vi "Create Name.vi"(6 "Name":string, 8 "error in":errorcluster, 9 "Name Library File Path":path, 10 "Active Project":refnum<vi>) -> (0 "error out":errorcluster, 2 "Name":T1)   [LabVIEW 2020, in "_Rescript.lvlib" / "Msg.lvlib" / "Msg.lvclass"]
uses:
  Msg.lvclass
  Name.ctl
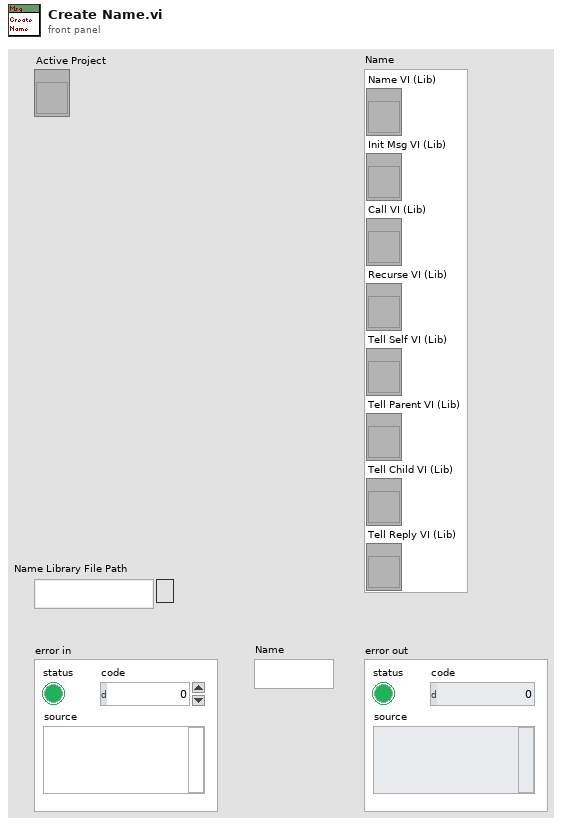
[diagram p1: front panel]
types:
  T1 = typedef "_Rescript.lvlib/Msg.lvlib/Msg.lvclass/Name.ctl" = cluster{"Name VI (Lib)":refnum<vi>, "Init Msg VI (Lib)":refnum<vi>, "Call VI (Lib)":refnum<vi>, "Recurse VI (Lib)":refnum<vi>, "Tell Self VI (Lib)":refnum<vi>, "Tell Parent VI (Lib)":refnum<vi>, "Tell Child VI (Lib)":refnum<vi>, "Tell Reply VI (Lib)":refnum<vi>}
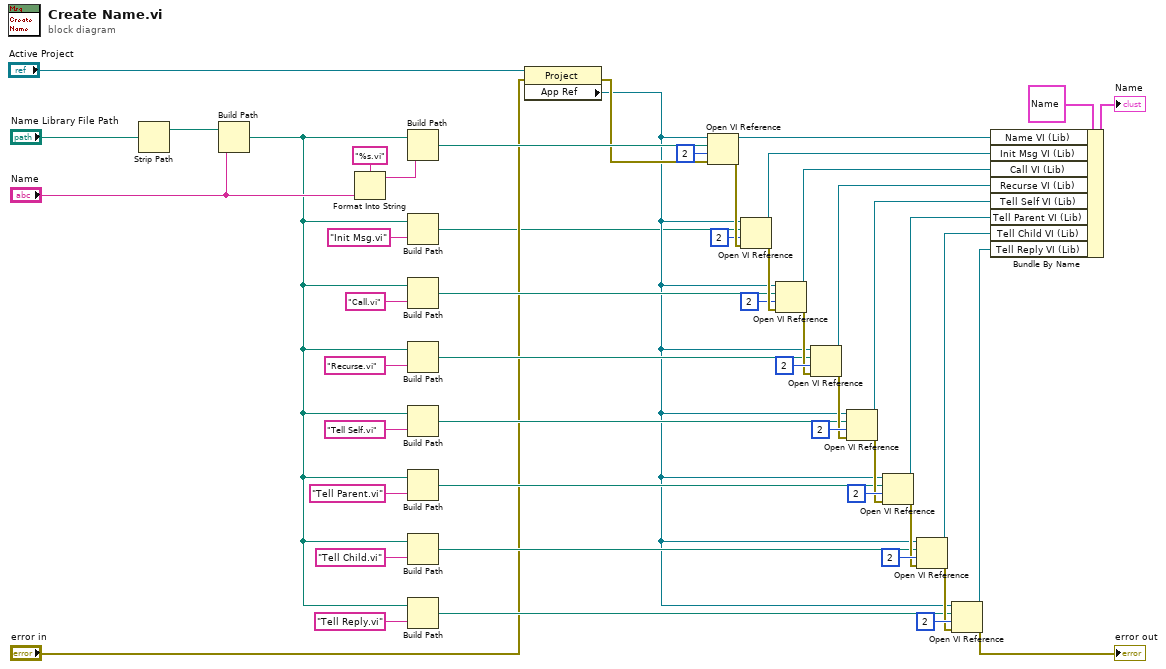
[diagram p0: block diagram]
diagram:
  n1 = Strip Path(path="Name Library File Path") -> (stripped path=w8:path)  [unwired: 1 out]
  n2 = Build Path(base path=w8, name or relative path="Name") -> (appended path=w6:path)
  n3 = Format Into String(format string="%s.vi", "Name") -> (resulting string=w48:string)  [unwired: 2 in, 1 out]
  n4 = Build Path(base path=w6, name or relative path=w48) -> (appended path=w47:path)
  n5 = Build Path(base path=w6, name or relative path="Init Msg.vi" ("format string")) -> (appended path=w2:path)
  n6 = Build Path(base path=w6, name or relative path="Call.vi" ("format string")) -> (appended path=w30:path)
  n7 = Build Path(base path=w6, name or relative path="Recurse.vi" ("format string")) -> (appended path=w29:path)
  n8 = Build Path(base path=w6, name or relative path="Tell Self.vi" ("format string")) -> (appended path=w28:path)
  n9 = Build Path(base path=w6, name or relative path="Tell Parent.vi" ("format string")) -> (appended path=w27:path)
  n10 = Build Path(base path=w6, name or relative path="Tell Child.vi" ("format string")) -> (appended path=w26:path)
  n11 = Build Path(base path=w6, name or relative path="Tell Reply.vi" ("format string")) -> (appended path=w21:path)
  n12 = property class="Project"(reference="Active Project", error in="error in") -> (error out=w10:errorcluster, "App Ref"=w3:refnum<vi>)  [unwired: 1 out]
  n13 = Open VI Reference(application reference (local)=w3, vi path=w47, options=2, error in (no error)=w10) -> (vi reference=w9:refnum<vi>, error out=w51:errorcluster)  [unwired: 2 in]
  n14 = Open VI Reference(application reference (local)=w3, vi path=w2, options=2, error in (no error)=w51) -> (vi reference=w1:refnum<vi>, error out=w50:errorcluster)  [unwired: 2 in]
  n15 = Open VI Reference(application reference (local)=w3, vi path=w30, options=2, error in (no error)=w50) -> (vi reference=w18:refnum<vi>, error out=w39:errorcluster)  [unwired: 2 in]
  n16 = Open VI Reference(application reference (local)=w3, vi path=w29, options=2, error in (no error)=w39) -> (vi reference=w17:refnum<vi>, error out=w38:errorcluster)  [unwired: 2 in]
  n17 = Open VI Reference(application reference (local)=w3, vi path=w28, options=2, error in (no error)=w38) -> (vi reference=w16:refnum<vi>, error out=w37:errorcluster)  [unwired: 2 in]
  n18 = Open VI Reference(application reference (local)=w3, vi path=w27, options=2, error in (no error)=w37) -> (vi reference=w15:refnum<vi>, error out=w36:errorcluster)  [unwired: 2 in]
  n19 = Open VI Reference(application reference (local)=w3, vi path=w26, options=2, error in (no error)=w36) -> (vi reference=w14:refnum<vi>, error out=w23:errorcluster)  [unwired: 2 in]
  n20 = Open VI Reference(application reference (local)=w3, vi path=w21, options=2, error in (no error)=w23) -> (vi reference=w13:refnum<vi>, error out=→"error out":errorcluster)  [unwired: 2 in]
  n21 = Bundle By Name(cluster=T1 {"Name VI (Lib)"=refnum, "Init Msg VI (Lib)"=refnum, "Call VI (Lib)"=refnum, "Recurse VI (Lib)"=refnum, "Tell Self VI (Lib)"=refnum, "Tell Parent VI (Lib)"=refnum, "Tell Child VI (Lib)"=refnum, "Tell Reply VI (Lib)"=refnum} ("VI Refs"), "Name VI (Lib)"=w9, "Init Msg VI (Lib)"=w1, "Call VI (Lib)"=w18, "Recurse VI (Lib)"=w17, "Tell Self VI (Lib)"=w16, "Tell Parent VI (Lib)"=w15, "Tell Child VI (Lib)"=w14, "Tell Reply VI (Lib)"=w13) -> (→"Name":T1)
